vi "output_scaling_factor.vi"(11 "which clamp":enum16{"VClamp", "IClamp"}(ring)) -> (3 "output scaling factor":dbl)   [LabVIEW 2019]
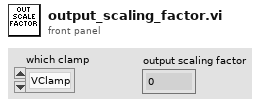
[diagram p1: front panel]
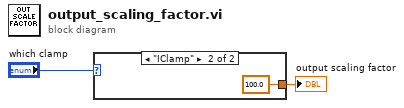
[diagram p0: block diagram]
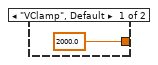
[diagram p2: hidden frame]
diagram:
  n1 = case shown="\"IClamp\"" "which clamp" {
    tunnel: [2000.0 100.0] -> w1
    frame "VClamp", Default {
    }
    frame "IClamp" {
    }
  }
  "output scaling factor" <- w1
